vi "AB_Engine_Update_Paths_In_Palette_Data.vi"(0 "palette data in":T1={"display name"="", "view format"=2, "palette width"=0, "items"=[], "256 color icon"=bytes[0], "B&W color icon"=bytes[0], "help information"={"help tag"="", "help file path "=path ""}, "palette description"="", "synchronize information"={"synchronize with directory"=FALSE, "synchronize directory path"=path ""}} {"view format" items=["Icons", "Text", "Icons and Text"]}, 5 "old paths":path[](array[path]), 7 "new paths":path[](array[path]), 9 "old dir paths":path[](array[path]), 11 "new dir paths":path[](array[path])) -> (4 "palette data out":T1={"display name"="", "view format"=2, "palette width"=0, "items"=[], "256 color icon"=bytes[0], "B&W color icon"=bytes[0], "help information"={"help tag"="", "help file path "=path ""}, "palette description"="", "synchronize information"={"synchronize with directory"=FALSE, "synchronize directory path"=path ""}} {"view format" items=["Icons", "Text", "Icons and Text"]})   [LabVIEW 2020]
uses:
  <vilib>/Palette API/Palette Menu/Public Type Define/Palette Data.ctl
  <vilib>/Palette API/Palette Menu/Public Type Define/View Format.ctl
  <vilib>/Palette API/Palette Menu/Public Type Define/Items.ctl
  <vilib>/Palette API/Palette Menu/Public Type Define/Item.ctl
  <vilib>/Palette API/Palette Menu/Public Type Define/Help Info.ctl
  <vilib>/Palette API/Palette Menu/Public Type Define/Synchronize Info.ctl
  <vilib>/Palette API/Palette Menu/Palette Menu.lvlib
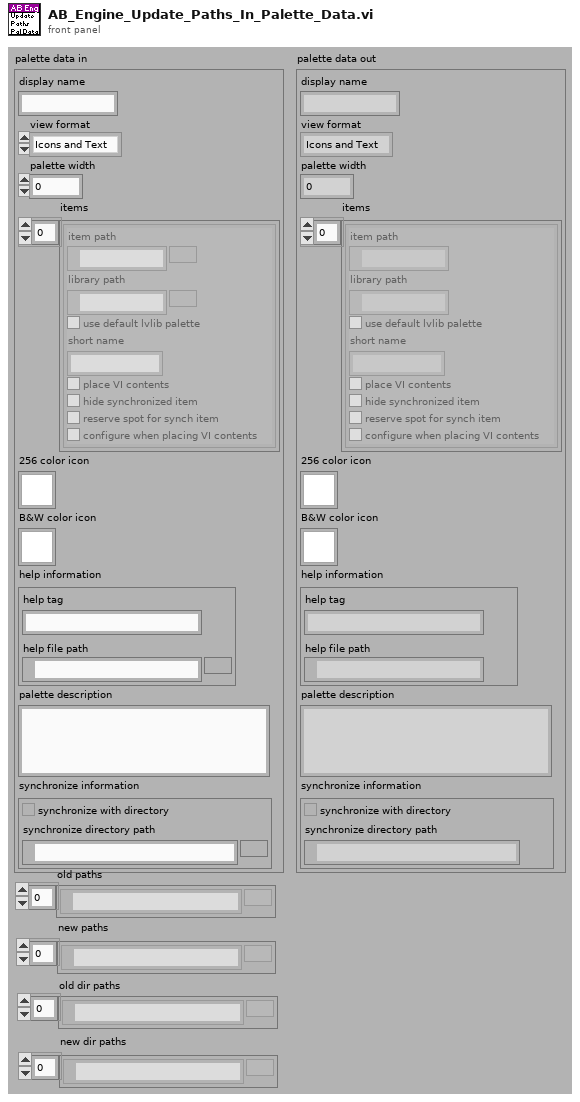
[diagram p1: front panel]
types:
  T1 = typedef "Palette Menu.lvlib/Palette Data.ctl" = cluster{"display name":string, "view format":T2, "palette width":i16, "items":T3, "256 color icon":picture, "B&W color icon":picture, "help information":T5, "palette description":string, "synchronize information":T6}
  T2 = typedef "Palette Menu.lvlib/View Format.ctl" = u16
  T3 = typedef "Palette Menu.lvlib/Items.ctl" = T4[]
  T4 = typedef "Palette Menu.lvlib/Item.ctl" = cluster{"item path":path, "library path":path, "use default lvlib palette":bool, "short name":string, "place VI contents":bool, "hide synchronized item":bool, "reserve spot for synch item":bool, "configure when placing VI contents":bool}
  T5 = typedef "Palette Menu.lvlib/Help Info.ctl" = cluster{"help tag":string, "help file path ":path}
  T6 = typedef "Palette Menu.lvlib/Synchronize Info.ctl" = cluster{"synchronize with directory":bool, "synchronize directory path":path}
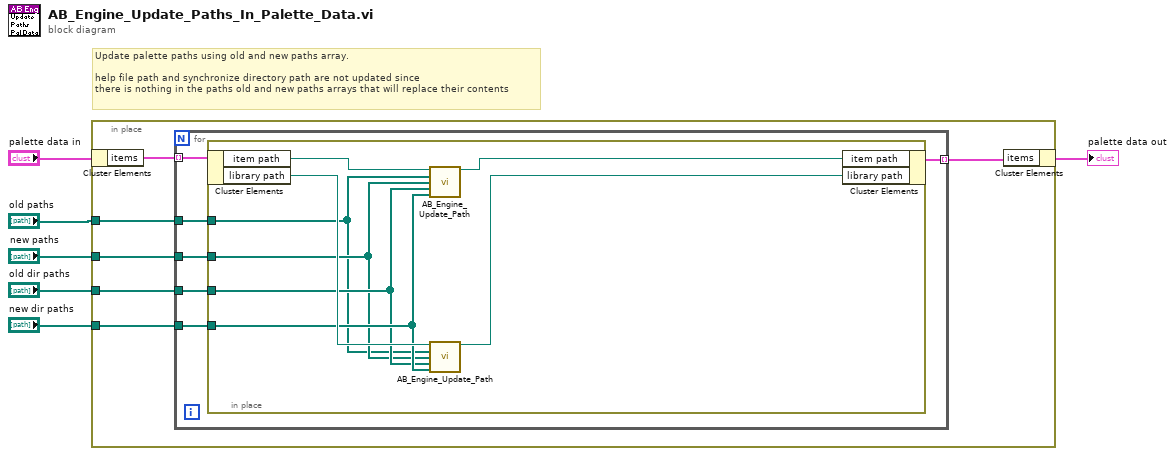
[diagram p0: block diagram]
diagram:
  # "Update palette paths using old and new paths array.\n\nhelp file path and synchronize directory path are not updated since \nthere is nothing in the paths old and new paths arrays that will replace their contents"
  n1 = in-place {
    in-place-border: "old paths" -> [w10]
    in-place-border: "new paths" -> [w9]
    in-place-border: "old dir paths" -> [w8]
    in-place-border: "new dir paths" -> [w7]
    n2 = in-place-cluster #1("palette data in") -> ("items"=w12:T3)
    n3 = for {
      tunnel: w12 -> [w18] mode=indexing
      tunnel: [w17] -> w11 mode=indexing
      tunnel: w10 -> [w16]
      tunnel: w9 -> [w15]
      tunnel: w8 -> [w14]
      tunnel: w7 -> [w13]
      n4 = in-place {
        in-place-border: w16 -> [w19]
        in-place-border: w15 -> [w20]
        in-place-border: w14 -> [w21]
        in-place-border: w13 -> [w22]
        n5 = in-place-cluster #2(w18) -> ("item path"=w26:path, "library path"=w25:path)
        n6 = call <vilib>:"AB_Engine_Update_Path.vi"("old path"=w26, "old paths"=w19, "new paths"=w20, "old dir paths"=w21, "new dir paths"=w22) -> ("new path"=w24:path)  [unwired: 10 in]
        n7 = call <vilib>:"AB_Engine_Update_Path.vi"("old path"=w25, "old paths"=w19, "new paths"=w20, "old dir paths"=w21, "new dir paths"=w22) -> ("new path"=w23:path)  [unwired: 10 in]
        n8 = in-place-cluster #2("item path"=w24, "library path"=w23) -> (w17:T4)
      }
    }
    n9 = in-place-cluster #1("items"=w11) -> (→"palette data out":T1)
  }
